vi "StackFromSingleWithPayload.vi"(6 "Payload":variant, 9 "Action":string) -> (1 "Stack out":refnum<class "Stack.lvclass">)   [LabVIEW 2024, in "ActionStack.lvlib" / "Stack.lvclass"]
uses:
  Stack.lvclass
  Stack.lvclass/Stack.ctl
  Action/SingleWithPayload.vi
  Action/Action.lvclass
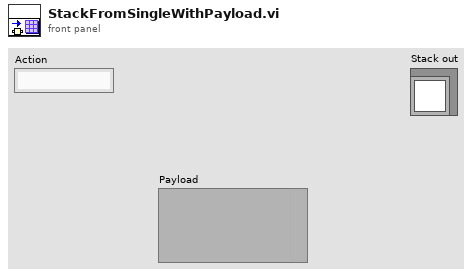
[diagram p1: front panel]
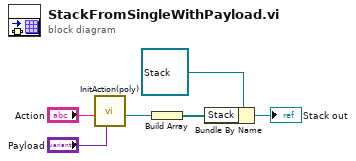
[diagram p0: block diagram]
diagram:
  n1 = call-poly "InitAction(poly).vi"("Payload"="Payload", "Action"="Action") -> ("ActionStack out"=w2:refnum<class "Action.lvclass">)  [unwired: 9 in]
  n2 = Build Array(w2) -> (w5:refnum<class "Action.lvclass">[])
  n3 = Bundle By Name(cluster=refnum<class "Stack.lvclass"> refnum ("ActionStack.lvclass"), "Stack"=w5) -> (→"Stack out":refnum<class "Stack.lvclass">)
